vi "new.vi"(8 "error in (no error)":errorcluster, 10 "stopMessage":string, 11 "msgUserEvent":refnum<user-event>) -> (0 "error out":errorcluster, 3 "MsgUserEventStopMechanism Out":refnum<class "MsgUserEventStopMechanism.lvclass">)   [LabVIEW 2023, in "TLC_Daemon.lvlib" / "MsgUserEventStopMechanism.lvclass"]
doc: "Initializes the stop mechanism.\n_____________________________________\nTLC Daemon 1.0.0.2\nCopyright (c) 2026 Andrea Cadei"
uses:
  MsgUserEventStopMechanism.lvclass
  MsgUserEventStopMechanism.lvclass/MsgUserEventStopMechanism.ctl
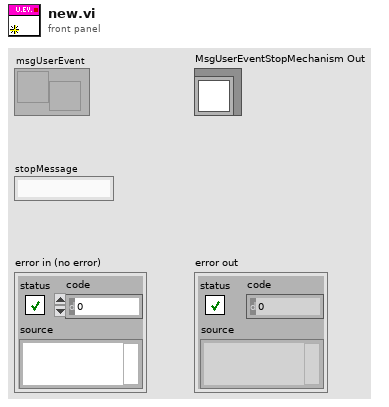
[diagram p1: front panel]
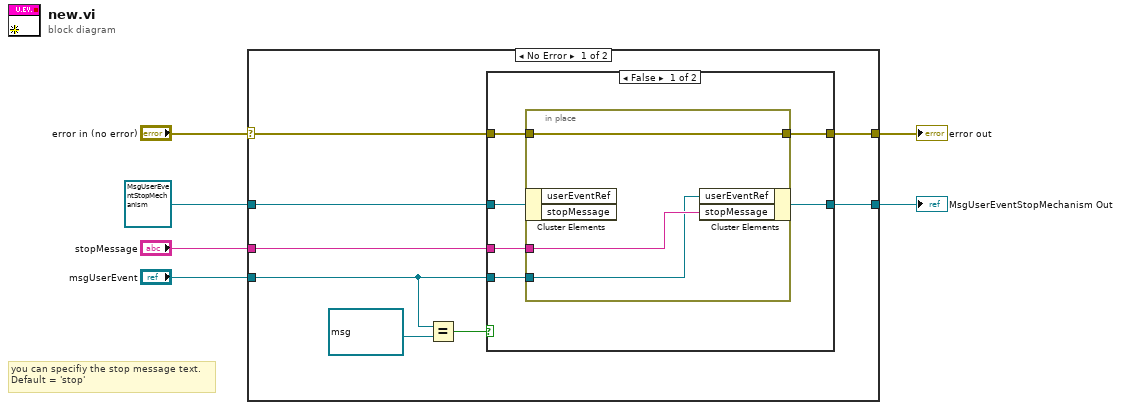
[diagram p0: block diagram]
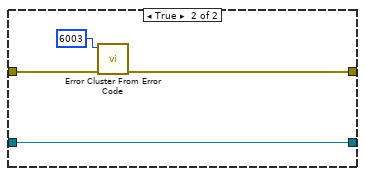
[diagram p2: hidden frame]
diagram:
  # "you can specifiy the stop message text.\nDefault = 'stop'"
  n1 = case shown="No Error" "error in (no error)" {
    selector: "error in (no error)" -> [w10 w29]
    tunnel: [w14 w29] -> w6
    tunnel: [w13 w28] -> w3
    tunnel: refnum<class "MsgUserEventStopMechanism.lvclass"> refnum ("MsgUserEventStopMechanism In") -> [w11 w28]
    tunnel: "stopMessage" -> [w12 _]
    tunnel: "msgUserEvent" -> [w9 _]
    frame No Error {
      n2 = Equal?(x=w9, y=refnum<user-event> refnum ("x")) -> (x = y?=w7:bool)
      n3 = case shown="False" w7 {
        tunnel: [w20 w26] -> w14
        tunnel: [w19 w25] -> w13
        tunnel: w12 -> [w18 _]
        tunnel: w11 -> [w17 w25]
        tunnel: w10 -> [w16 w24]
        tunnel: w9 -> [w15 _]
        frame False {
          n4 = in-place {
            in-place-border: w16 -> [w23]
            in-place-border: [w23] -> w20
            in-place-border: w18 -> [w22]
            in-place-border: w15 -> [w21]
            n5 = in-place-cluster #1(w17) -> ()  [unwired: 2 out]
            n6 = in-place-cluster #1("userEventRef"=w21, "stopMessage"=w22) -> (w19:refnum<class "MsgUserEventStopMechanism.lvclass">)
          }
        }
        frame True {
          n7 = call <vilib>:"Error Cluster From Error Code.vi"("error in (no error)"=w24, "error code (0)"=6003) -> ("error out"=w26:errorcluster)  [unwired: 7 in]
        }
      }
    }
    frame Error {
    }
  }
  "error out" <- w6
  "MsgUserEventStopMechanism Out" <- w3
